vi "Write.vi"(8 "error in (no error)":errorcluster, 10 "write buffer":string, 11 "Serial in":refnum<class "Serial.lvclass">) -> (0 "error out":errorcluster, 2 "return count":u32, 3 "Serial out":refnum<class "Serial.lvclass">)   [LabVIEW 2020, in "Serial.lvclass"]
uses:
  Serial.lvclass
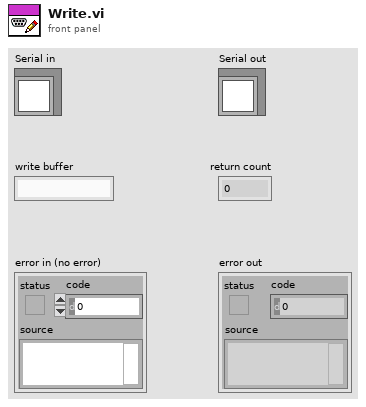
[diagram p1: front panel]
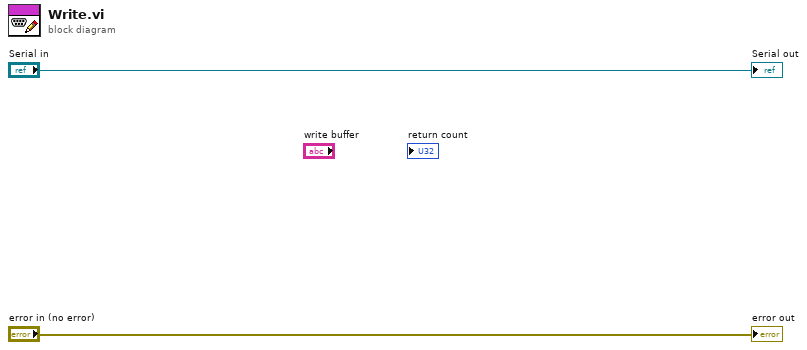
[diagram p0: block diagram]
diagram:
  "error out" <- "error in (no error)"
  "Serial out" <- "Serial in"
